vi "Reset_Instr.vi"(8 "error in (no error)":errorcluster caption="entrée d'erreur (pas d'erreur)", 11 "Class Relay_Board en entrée":refnum<class "Class Instrument UART.lvclass">) -> (0 "error out":errorcluster caption="sortie d'erreur", 3 "Class Relay_Board en Sortie":refnum<class "Class Instrument UART.lvclass">)   [LabVIEW 2020, in "Library Instrument & Equipement.lvlib" / "Library Instruments.lvlib" / "Class Instrument UART.lvclass"]
uses:
  Class Instrument UART.lvclass
  Class Instrument UART.lvclass/Class Instrument UART.ctl
  Instrument (Default)/Class Instrument (Default).lvclass
  UART/UART (Default)/Class UART (Default).lvclass
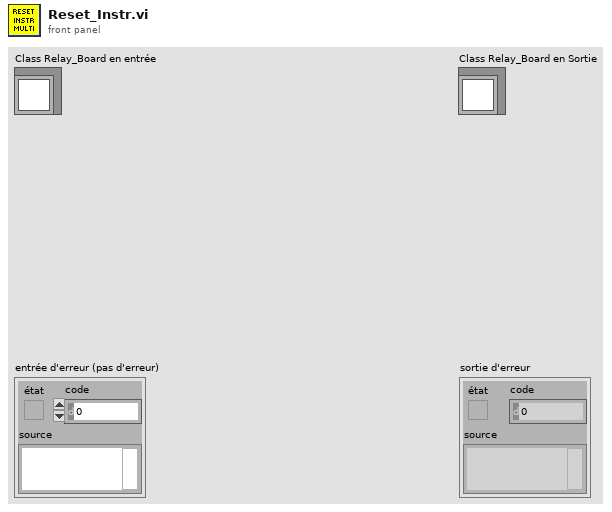
[diagram p1: front panel]
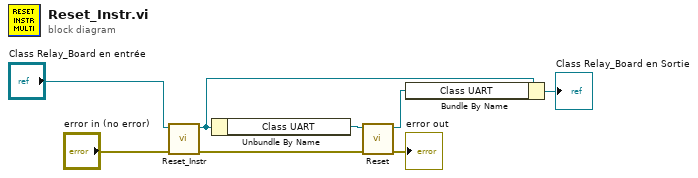
[diagram p0: block diagram]
diagram:
  n1 = call-parent "Reset_Instr.vi"("error in (no error)"="error in (no error)", "Class Instrument (Default) en entrée"="Class Relay_Board en entrée") -> ("error out"=w4:errorcluster, "Class Instrument (Default) en sortie"=w5:refnum<class "Class Instrument UART.lvclass">)  [unwired: 8 in]
  n2 = Unbundle By Name(w5) -> ("Class UART"=w2:refnum<class "Class UART (Default).lvclass">)
  n3 = call-dynamic "Reset.vi"("error in (no error)"=w4, "Class UART (Default) en entrée"=w2) -> ("error out"=→"error out":errorcluster, "Class UART (Default) en sortie"=w1:refnum<class "Class UART (Default).lvclass">)  [unwired: 8 in]
  n4 = Bundle By Name(cluster=w5, "Class UART"=w1) -> (→"Class Relay_Board en Sortie":refnum<class "Class Instrument UART.lvclass">)
